vi "Destroy.vi"(6 "Save Instruments?(F)":bool, 8 "error in (no error)":errorcluster, 9 "Auto Save(T)":bool=TRUE, 11 "CSM-Helper in":refnum<class "CSM-Helper.lvclass">) -> (0 "error out":errorcluster, 3 "CSM-Helper out":refnum<class "CSM-Helper.lvclass">)   [LabVIEW 2017, in "CSM-Helper.lvclass"]
doc: "### Destroy.vi\n\n-- <b>Controls</b> --\n- <b>Save Instruments?(F)</b>:\n- <b>CSM-Helper in</b>: CSMHelper input\n\n-- <b>Indicators</b> --\n- <b>CSM-Helper out</b>: CSMHelper output"
uses:
  CSM-Helper.lvclass
  CSM-Helper.lvclass/CSM-Helper.ctl
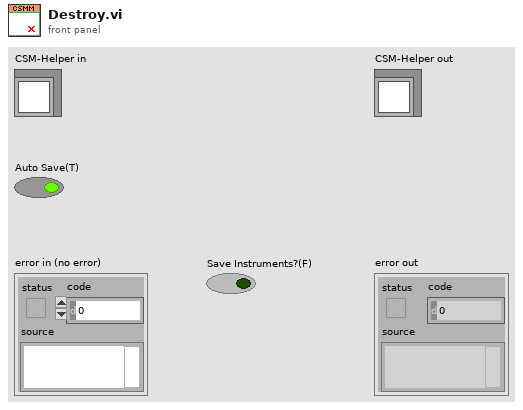
[diagram p1: front panel]
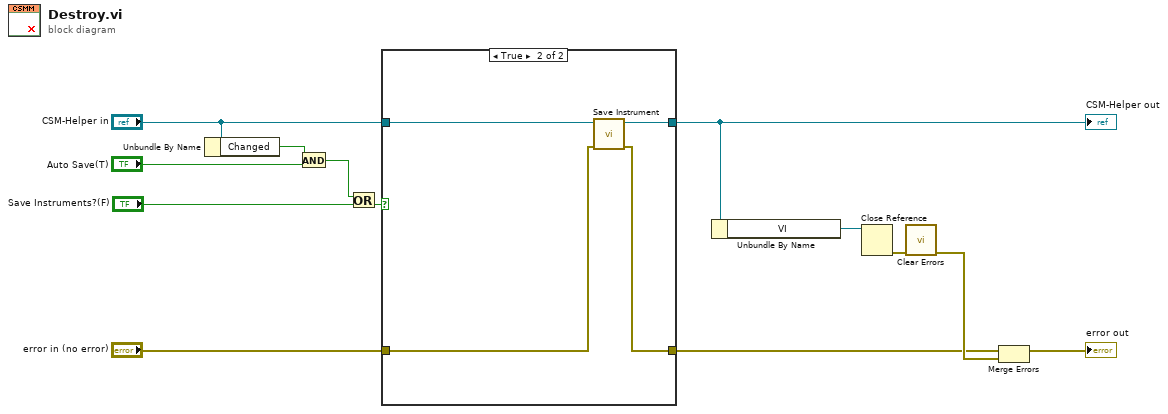
[diagram p0: block diagram]
diagram:
  n1 = Unbundle By Name("CSM-Helper in") -> ("Changed"=w1:bool)
  n2 = And(x=w1, y="Auto Save(T)") -> (x .and. y?=w3:bool)
  n3 = Or(x=w3, y="Save Instruments?(F)") -> (x .or. y?=w5:bool)
  n4 = case shown="True" w5 {
    tunnel: "CSM-Helper in" -> [w14 w19]
    tunnel: [w14 w18] -> w9
    tunnel: "error in (no error)" -> [w15 w17]
    tunnel: [w15 w16] -> w7
    frame False {
    }
    frame True {
      n5 = call "Save Instrument.vi"("error in (no error)"=w17, "CSM-Helper in"=w19) -> ("error out"=w16:errorcluster, "CSM-Helper out"=w18:refnum<class "CSM-Helper.lvclass">)  [unwired: 8 in]
    }
  }
  "CSM-Helper out" <- w9
  n6 = Unbundle By Name(w9) -> ("VI"=w13:refnum<vi>)
  n7 = Close Reference(reference=w13) -> (error out=w12:errorcluster)  [unwired: 1 in]
  n8 = call <vilib>:"Clear Errors.vi"("error in (no error)"=w12) -> ("error out"=w10:errorcluster)  [unwired: 5 in, 1 out]
  n9 = Merge Errors(w7, w10) -> (→"error out":errorcluster)
